vi "Split String.vi"(0 "split ([ \\t]+)":string="[ \\t]+", 1 "lower":bool, 4 "string":string) -> (2 "found split?":bool, 3 "after split":string, 6 "before empty?":bool, 7 "before split":string)   [LabVIEW 2009, in "Tools_String.lvlib"]
uses:
  Tools_String.lvlib
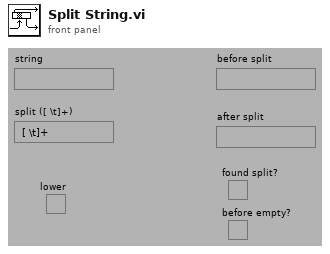
[diagram p1: front panel]
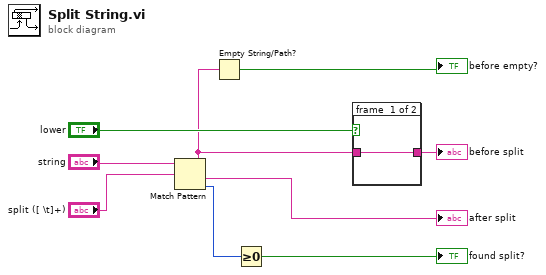
[diagram p0: block diagram]
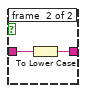
[diagram p2: hidden frame]
diagram:
  n1 = Match Pattern(string="string", regular expression="split ([ \\t]+)") -> (before substring=w2:string, after substring=→"after split":string, offset past match=w6:i32)  [unwired: 2 out]
  n2 = Empty String/Path?(string/path=w2) -> (empty?=→"before empty?":bool)
  n3 = Greater Or Equal To 0?(x=w6) -> (x >= 0?=→"found split?":bool)
  n4 = case shown="True" "lower" {
    tunnel: w2 -> [w10 w12]
    tunnel: [w10 w11] -> w1
    frame #0 {
    }
    frame #1 {
      n5 = To Lower Case(string=w12) -> (all lower case string=w11:string)
    }
  }
  "before split" <- w1
